vi "xiC - FormatPRMToTree.vi"(7 "PRM[]":T1[](array[typedef]), 8 "error in (no error)":errorcluster, 9 "SectionName":string, 11 "Attributes":T2) -> (0 "error out":errorcluster, 3 "Attributes Out":T2, 4 "TreeItems[]":T4(array[cluster]))   [LabVIEW 2015]
uses:
  xiCamLib/xiLIB/Typedefs/xiLIB - PRM_Function.ctl
  C:/GIT/Cameras3.x/Integrations/Labview/xiLib/xiLIB_32bit/xiLIB/xiCamLib/API/x86/xiApi.NET.dll
  xiLIB_32bit/xiLIB/xiCamLib/API/x86/xiApi.NET.dll
  xiC - TreeDisplayType.ctl
  xiC - Attributes.ctl
  xiCamLib/xiCam/PRM/PRM/PRM_v2.ctl
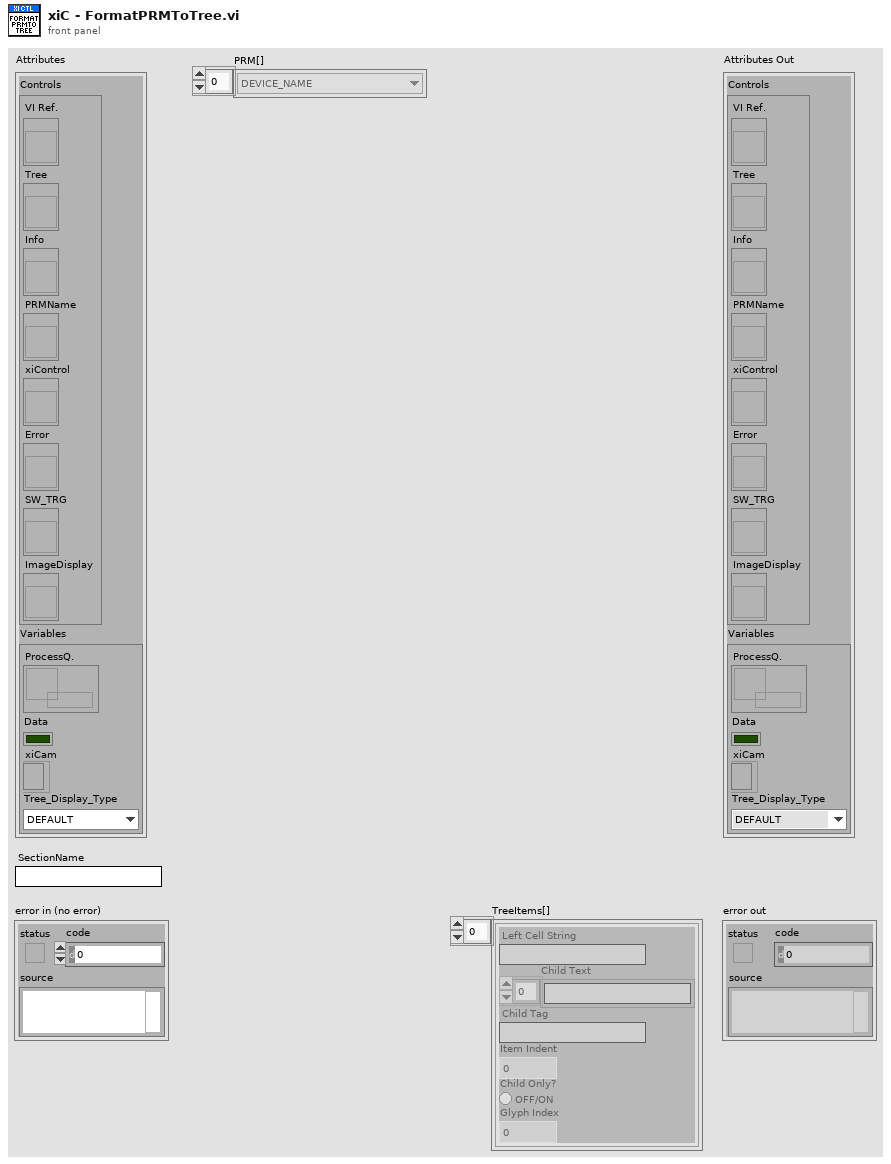
[diagram p1: front panel]
types:
  T1 = typedef "PRM_v2.ctl" = enum16{"ACQ_BUFFER_SIZE", "ACQ_FRAME_BURST_COUNT", "ACQ_TIMING_MODE", "ACQ_TRANSPORT_BUFFER_SIZE", "AE_MAX_LIMIT", "AEAG", "AEAG_LEVEL", "API_VERSION", "AG_MAX_LIMIT", "APPLY_CMS", "AUTO_BANDWIDTH_CALCULATION", "AUTO_WB", "AVAILABLE_BANDWIDTH", "AVAILABLE_BANDWIDTH_MAX", "AVAILABLE_BANDWIDTH_MIN", "BPC", "BUFFER_POLICY", "BUFFERS_QUEUE_SIZE", "CC_MATRIX_00", "CC_MATRIX_01", "CC_MATRIX_02", "CC_MATRIX_03", "CC_MATRIX_10", "CC_MATRIX_11", "CC_MATRIX_12", "CC_MATRIX_13", "CC_MATRIX_20", "CC_MATRIX_21", "CC_MATRIX_22", "CC_MATRIX_23", "CC_MATRIX_30", "CC_MATRIX_31", "CC_MATRIX_32", "CC_MATRIX_33", "CHIP_TEMP", "CMS", "COLOR_FILTER_ARRAY", "COOLING", "DEBOUNCE_EN", "DEBOUNCE_POL", "DEBOUNCE_T0", "DEBOUNCE_T1", "DEBUG_LEVEL", "DEFAULT_CC_MATRIX", "DEVICE_INSTANCE_PATH", "DEVICE_MODEL_ID", "DEVICE_NAME", "DEVICE_SN", "DEVICE_TYPE", "DEVICE_USER_ID", "DOWNSAMPLING", "DOWNSAMPLING_MAX", "DOWNSAMPLING_MIN", "DOWNSAMPLING_TYPE", "DRV_VERSION", "EXP_PRIORITY", "EXPOSURE", "EXPOSURE_DIRECT_UPDATE", "EXPOSURE_MAX", "EXPOSURE_MIN", "FFS_FILE_NAME", "FPGA1_VERSION", "FRAMERATE", "FRAMERATE_MAX", "FRAMERATE_MIN", "FREE_FFS_SIZE", "GAIN", "GAIN_DIRECT_UPDATE", "GAIN_MAX", "GAIN_MIN", "GAMMAC", "GAMMAY", "GPI_LEVEL", "GPI_MODE", "GPI_SELECTOR", "GPI_SELECTOR_MAX", "GPI_SELECTOR_MIN", "GPO_MODE", "GPO_SELECTOR", "GPO_SELECTOR_MAX", "GPO_SELECTOR_MIN", "HDR", "HDR_T1", "HDR_T2", "HEIGHT", "HEIGHT_MAX", "HEIGHT_MIN", "HOUSE_TEMP", "IMAGE_DATA_FORMAT", "IMAGE_IS_COLOR", "INPUT_CMS_PROFILE", "IS_COOLED", "IS_DEVICE_EXIST", "KNEEPOINT1", "KNEEPOINT2", "LED_MODE", "LED_SELECTOR", "LED_SELECTOR_MAX", "LED_SELECTOR_MIN", "LIMIT_BANDWIDTH", "LIMIT_BANDWIDTH_MAX", "LIMIT_BANDWIDTH_MIN", "LUT_EN", "LUT_INDEX", "LUT_INDEX_MAX", "LUT_INDEX_MIN", "LUT_VALUE", "LUT_VALUE_MAX", "LUT_VALUE_MIN", "MANUAL_WB", "MCU1_VERSION", "MCU2_VERSION", "OFFSET_X", "OFFSET_X_MAX", "OFFSET_X_MIN", "OFFSET_Y", "OFFSET_Y_MAX", "OFFSET_Y_MIN", "OUTPUT_CMS_PROFILE", "OUTPUT_DATA_BIT_DEPTH", "OUTPUT_DATA_PACKING", "READ_FILE_FFS", "RECENT_FRAME", "SENSOR_DATA_BIT_DEPTH", "SENSOR_MODE", "SENSOR_TAPS", "SHARPNESS", "SHUTTER_TYPE", "TARGET_TEMP", "TRG_DELAY", "TRG_SELECTOR", "TRG_SOFTWARE", "TRG_SOURCE", "USED_FFS_SIZE", "WB_KB", "WB_KG", "WB_KR", "WIDTH", "WIDTH_MAX", "WIDTH_MIN", "WRITE_FILE_FFS", "ACQ_BUFFER_SIZE_UNIT", "ACQ_TRANSPORT_BUFFER_COMMIT", "AEAG_ROI_HEIGHT", "AEAG_ROI_OFFSET_X", "AEAG_ROU_OFFSET_Y", "AEAG_ROI_WIDTH", "API_CONTEXT_LIST", "BINNING_HORIZONTAL", "BINNING_SELECTOR", "BINNING_VERTICAL", "COLUMN_FPN_CORRECTION", "COUNTER_SELECTOR", "COUNTER_VALUE", "DECIMATION_HORIZONTAL", "DECIMATION_SELECTOR", "DECIMATION_VERTICAL", "DEVICE_ID", "DEVICE_LOCATION_PATH", "DEVICE_MANIFEST", "DEVICE_RESET", "DEVICE_SENS_SN", "EXPOSURE_BURST_COUNT", "FFS_ACCESS_KEY", "GAIN_SELECTOR", "HW_REVISION", "IMAGE_BLACK_LEVEL", "IMAGE_DATA_BIT_DEPTH", "IMAGE_DATA_FORMAT_RGB32_ALPHA", "IMAGE_PAYLOAD_SIZE", "LENS_APERTURE_VALUE", "LENS_FEATURE", "LENS_FEATURE_SELECTOR", "LENS_FOCAL_LENGTH", "LENS_FOCUS_DISTANCE", "LENS_FOCUS_MOVE", "LENS_FOCUS_MOVEMENT_VALUE", "LENS_MODE", "OUTPUT_DATA_PACKING_TYPE", "SENSOR_CLOCK_FREQ_HZ", "SENSOR_CLOCK_FREQ_INDEX", "SENSOR_FEATURE_SELECTOR", "SENSOR_FEATURE_VALUE", "SENSOR_OUTPUT_CHANNEL_COUNT", "TRANSPORT_PIXEL_FORMAT", "TS_RST_MODE", "TS_RST_SOURCE"}
  T2 = typedef "xiC - Attributes.ctl" = cluster{"Controls":cluster{"VI Ref.":refnum<vi>, "Tree":refnum<vi>, "Info":refnum<vi>, "PRMName":refnum<vi>, "xiControl":refnum<vi>, "Error":refnum<vi>, "SW_TRG":refnum<vi>, "ImageDisplay":refnum<vi>}, "Variables":cluster{"ProcessQ.":refnum<queue>, "Data":bool, "xiCam":refnum<k24>, "Tree_Display_Type":T3}}
  T3 = typedef "xiC - TreeDisplayType.ctl" = enum16{"DEFAULT", "HIDE_MAX_MIN"}
  T4 = cluster{"Left Cell String":string, "Child Text":string[], "Child Tag":string, "Item Indent":i32, "Child Only?":bool, "Glyph Index":i32}[]
  T5 = cluster{"Left Cell String":string, "Child Text":string[], "Child Tag":string, "Item Indent":i32, "Child Only?":bool, "Glyph Index":i32}
  T6 = typedef "xiLIB - PRM_Function.ctl" = enum16{"Get / Set", "Get", "Set"}
  T7 = typedef "xiLIB - PRM_Attribute.ctl" = cluster{"Type":T8, "Method":T6, "Desc.":string, "PRM":T1}
  T8 = typedef "xiLIB - PRM_Type.ctl" = enum16{"Int32", "Float", "String", "DOWNSAMPLING_TYPE", "IMAGE_DATA_FORMAT", "BUFFER_POLICY", "TRG_SOURCE", "GPI", "GPO", "ACQ_TIMING_MODE", "BINNING_PATTERN", "BINNING_SELECTOR", "CMS_MODE", "COUNTER_SELECTOR", "DEBUG_LEVEL", "DECIMATION_PATTERN", "DECIMATION_SELECTOR", "GAIN_SELECTOR_TYPE", "LED_MODE", "LENS_FEATURE_SELECTOR", "LENS_MODE", "OUTPUT_DATA_PACKING_TYPE", "SENSOR_FEATURE_SELECTOR", "SHUTTER_TYPE", "TRG_SELECTOR", "TS_RST_MODE", "TS_RST_SOURCE"}
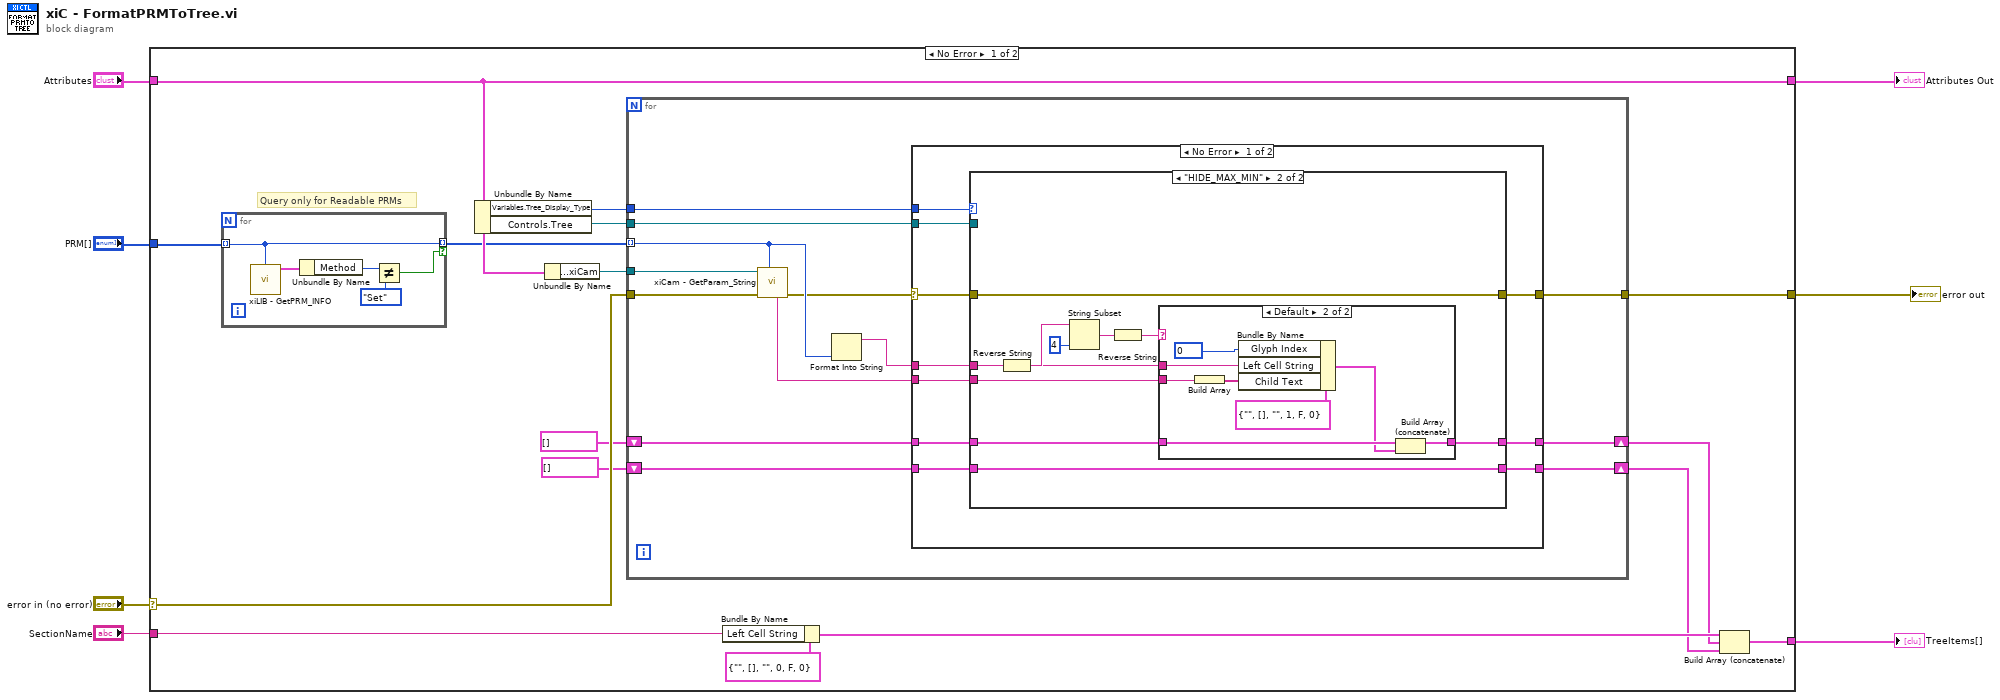
[diagram p0: block diagram]
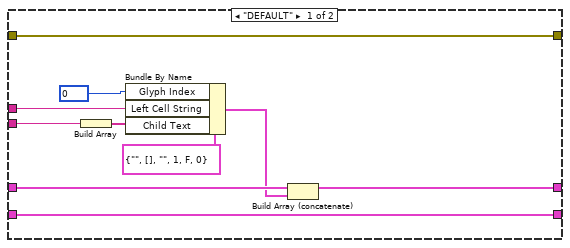
[diagram p2: hidden frame]
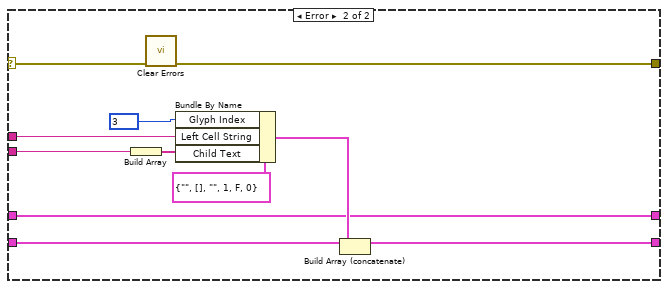
[diagram p4: hidden frame]
diagram:
  n1 = case shown="No Error" "error in (no error)" {
    selector: "error in (no error)" -> [w23 w93]
    tunnel: [w15 w93] -> w6
    tunnel: [w20 _] -> w5
    tunnel: "Attributes" -> [w19 w92]
    tunnel: [w19 w92] -> w3
    tunnel: "SectionName" -> [w18 _]
    tunnel: "PRM[]" -> [w9 _]
    frame No Error {
      # "Query only for Readable PRMs"
      n2 = for {
        tunnel: w9 -> [w25] mode=indexing
        tunnel: [w25] -> w8 mode=indexing if=w24
        n3 = call "xiLIB - GetPRM_INFO.vi"("PRM"=w25) -> ("PRM_Attributes"=w28:T7)  [unwired: 10 in]
        n4 = Unbundle By Name(w28) -> ("Method"=w27:T6)
        n5 = Not Equal?(x=w27, y=xiLIB_-_PRM_Function."Set") -> (x != y?=w24:bool)
      }
      n6 = Unbundle By Name(w19) -> ("Variables.Tree_Display_Type"=w13:T3, "Controls.Tree"=w14:refnum<vi>)
      n7 = Unbundle By Name(w19) -> ("Variables.xiCam"=w12:refnum<k24>)
      n8 = for {
        tunnel: w8 -> [w37] mode=indexing
        tunnel: w23 -> [w41]
        tunnel: w14 -> [w40]
        tunnel: w13 -> [w39]
        tunnel: w12 -> [w38]
        shift-right: [w30] -> w17
        shift-left: T4 [] -> [w33]
        shift-right: [w31] -> w16
        shift-left: T4 [] -> [w32]
        tunnel: [w34] -> w15
        n9 = call "xiCam - GetParam_String.vi"("PRM"=w37, "error in (no error)"=w41, "xiCam In"=w38) -> ("error out"=w36:errorcluster, "String_Value"=w35:string)  [unwired: 6 in, 1 out]
        n10 = Format Into String(w37) -> (resulting string=w29:string)  [unwired: 3 in, 1 out]
        n11 = case shown="No Error" w36 {
          selector: w36 -> [w48 w86]
          tunnel: w40 -> [w51 _]
          tunnel: w39 -> [w50 _]
          tunnel: [w49 w82] -> w34
          tunnel: w35 -> [w46 w88]
          tunnel: w29 -> [w47 w87]
          tunnel: w33 -> [w45 w81]
          tunnel: w32 -> [w43 w85]
          tunnel: [w42 w83] -> w31
          tunnel: [w44 w81] -> w30
          frame No Error {
            n12 = case shown="\"HIDE_MAX_MIN\"" w50 {
              tunnel: w51 -> [_ _]
              tunnel: w48 -> [w61 w71]
              tunnel: [w61 w71] -> w49
              tunnel: w47 -> [w57 w62]
              tunnel: w46 -> [w56 w70]
              tunnel: w45 -> [w55 w69]
              tunnel: [w53 w68] -> w44
              tunnel: w43 -> [w52 w67]
              tunnel: [w52 w67] -> w42
              frame "DEFAULT" {
                n13 = Build Array(w56) -> (w60:string[])
                n14 = Bundle By Name(cluster=T5 {"Left Cell String"="", "Child Text"=[], "Child Tag"="", "Item Indent"=1, "Child Only?"=FALSE, "Glyph Index"=0} ("Item"), "Glyph Index"=0, "Left Cell String"=w57, "Child Text"=w60) -> (w54:T5)
                n15 = Build Array (concatenate)(w55, w54) -> (w53:T4)
              }
              frame "HIDE_MAX_MIN" {
                n16 = Reverse String(1:w62) -> (0:w66:string)
                n17 = String Subset(string=w66, length (rest)=4 ("length (rest)")) -> (substring=w64:string)  [unwired: 1 in]
                n18 = Reverse String(1:w64) -> (0:w63:string)
                n19 = case shown="Default" w63 {
                  tunnel: w70 -> [_ w77]
                  tunnel: w69 -> [w72 w76]
                  tunnel: [w72 w74] -> w68
                  tunnel: w62 -> [_ w73]
                  frame "_MAX", "_MIN" {
                  }
                  frame Default {
                    n20 = Build Array(w77) -> (w80:string[])
                    n21 = Bundle By Name(cluster=T5 {"Left Cell String"="", "Child Text"=[], "Child Tag"="", "Item Indent"=1, "Child Only?"=FALSE, "Glyph Index"=0} ("Item"), "Glyph Index"=0, "Left Cell String"=w73, "Child Text"=w80) -> (w75:T5)
                    n22 = Build Array (concatenate)(w76, w75) -> (w74:T4)
                  }
                }
              }
            }
          }
          frame Error {
            n23 = Build Array(w88) -> (w91:string[])
            n24 = call <vilib>:"Clear Errors.vi"("error in (no error)"=w86) -> ("error out"=w82:errorcluster)  [unwired: 5 in, 1 out]
            n25 = Bundle By Name(cluster=T5 {"Left Cell String"="", "Child Text"=[], "Child Tag"="", "Item Indent"=1, "Child Only?"=FALSE, "Glyph Index"=0} ("Item"), "Glyph Index"=3, "Left Cell String"=w87, "Child Text"=w91) -> (w84:T5)
            n26 = Build Array (concatenate)(w85, w84) -> (w83:T4)
          }
        }
      }
      n27 = Bundle By Name(cluster=T5 {"Left Cell String"="", "Child Text"=[], "Child Tag"="", "Item Indent"=0, "Child Only?"=FALSE, "Glyph Index"=0} ("Item"), "Left Cell String"=w18) -> (w21:T5)
      n28 = Build Array (concatenate)(w21, w17, w16) -> (w20:T4)
    }
    frame Error {
    }
  }
  "error out" <- w6
  "TreeItems[]" <- w5
  "Attributes Out" <- w3
